vi "ts.vi"(7 "error in":errorcluster) -> (27 "error out":errorcluster)   [LabVIEW 2017]
uses:
  <vilib>/vision/NI_Vision_Development_Module.lvlib
panel:
  out "Image Out":T1(plugin-control)
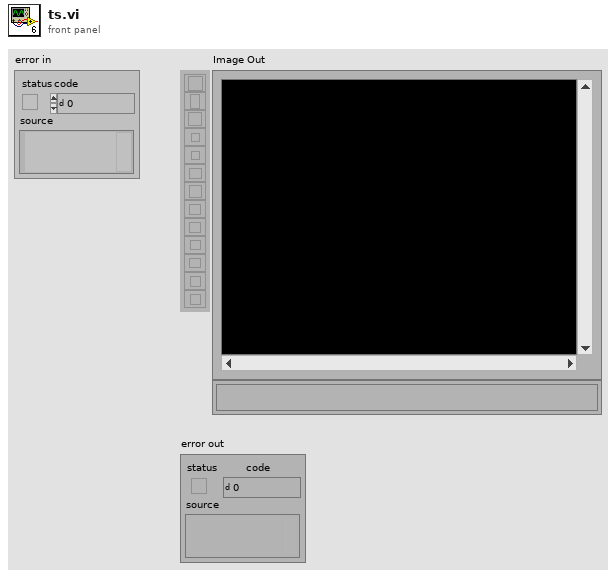
[diagram p1: front panel]
types:
  T1 = typedef "IMAQ Image.ctl" = refnum<image>
  T2 = cluster{"Origin Pixel":cluster{"X":sgl, "Y":sgl}, "Angle Relative to Horizontal (deg)":sgl, "Axis Reference":u32}
  T3 = typedef "Image Type" = u32
  T4 = cluster{"Origin Pixel":cluster{"X":sgl, "Y":sgl}, sgl, "Axis Reference":u32}
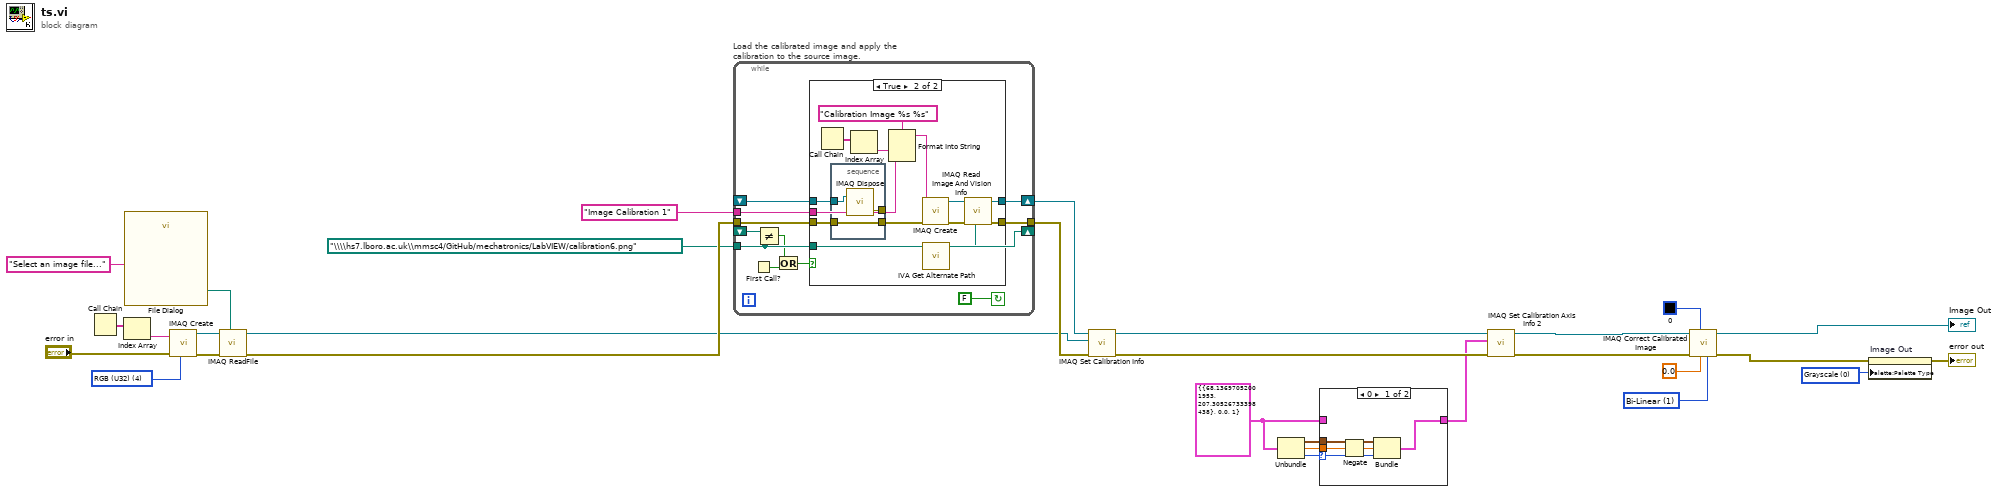
[diagram p0: block diagram]
diagram:
  w1 = u32 0 items=["Grayscale", "Binary", "Gradient", "Rainbow", "Temperature", "User Defined", "Binary 16 Bit", "Gradient 16 Bit", "Rainbow 16 Bit", "Temperature 16 Bit", "User Defined 16 Bit"] ("Palette Type")
  w8 = u32 1 items=["Zero Order", "Bi-Linear", "Quadratic", "Cubic Spline"] ("Interpolation Type")
  w12 = T2 {"Origin Pixel"={"X"=68.13697, "Y"=207.30527}, "Angle Relative to Horizontal (deg)"=0.0, "Axis Reference"=1} ("Calibration Axis Info")
  w22 = T3 4 items=["Grayscale (U8)", "Grayscale (I16)", "Grayscale (SGL)", "Complex (CSG)", "RGB (U32)", "HSL (U32)", "RGB (U64)", "Grayscale (U16)"] ("Image Type")
  n1 = Call Chain() -> (call chain=w26:string[])
  n2 = Index Array(array=w26) -> (element=w25:string)  [unwired: 1 in]
  n3 = call "File Dialog"("prompt"="Select an image file...") -> ("selected path"=w23:path)  [unwired: 6 in, 8 out]
  n4 = call "IMAQ Create"("Image Name"=w25, "Image Type"=w22, "error in (no error)"="error in") -> ("New Image"=w29:T1, "error out"=w28:errorcluster)  [unwired: 1 in, 1 out]
  n5 = call "IMAQ ReadFile"("File Path"=w23, "error in (no error)"=w28, "Image"=w29) -> ("error out"=w30:errorcluster, "Image Out"=w17:T1)  [unwired: 2 in, 5 out]
  n6 = while "Load the calibrated image and apply the calibration to the source image." {
    shift-right: [w41] -> w20
    shift-left: _ -> [w40]
    tunnel: [w38] -> w19
    tunnel: w30 -> [w37]
    tunnel: path "\\\\hs7.lboro.ac.uk\\mmsc4/GitHub/mechatronics/LabVIEW/calibration6.png" ("File Path") -> [w34]
    tunnel: "Image Calibration 1" ("Step Name") -> [w36]
    shift-right: [w34] -> _
    shift-left: _ -> [w35]
    stop <- FALSE continue-if-true
    n7 = First Call?() -> (First Call?: T/F=w33:bool)
    n8 = Not Equal?(x=w35, y=w34) -> (x != y?=w32:bool)
    n9 = Or(x=w32, y=w33) -> (x .or. y?=w31:bool)
    n10 = case shown="True" w31 {
      tunnel: [w43 w55] -> w41
      tunnel: w40 -> [w43 w47]
      tunnel: [w42 w52] -> w38
      tunnel: w37 -> [w42 w48]
      tunnel: w34 -> [_ w45]
      tunnel: w36 -> [_ w49]
      frame False {
      }
      frame True {
        n11 = Call Chain() -> (call chain=w51:string[])
        n12 = stacked-sequence {
          tunnel: w48 -> [w59]
          tunnel: w47 -> [w60]
          tunnel: [w59] -> w46
          tunnel: [w58] -> _
          frame #0 {
            n13 = call "IMAQ Dispose"("Image"=w60) -> ("error out"=w58:errorcluster)  [unwired: 2 in, 3 out]
          }
        }
        n14 = Index Array(array=w51) -> (element=w50:string)  [unwired: 1 in]
        n15 = Format Into String(format string="Calibration Image %s %s" ("Image Name"), w50, w49) -> (resulting string=w57:string)  [unwired: 2 in, 1 out]
        n16 = call "IMAQ Create"("Image Name"=w57, "error in (no error)"=w46) -> ("New Image"=w54:T1, "error out"=w53:errorcluster)  [unwired: 2 in, 1 out]
        n17 = call <vilib>:"IVA Get Alternate Path.vi"("Path In"=w45) -> ("Path Out"=w44:path)  [unwired: 10 out]
        n18 = call "IMAQ Read Image And Vision Info"("File Path"=w44, "error in (no error)"=w53, "Image"=w54) -> ("error out"=w52:errorcluster, "Image Out"=w55:T1)  [unwired: 1 in, 6 out]
      }
    }
  }
  n19 = call "IMAQ Set Calibration Info"("error in (no error)"=w19, "Image Dst"=w17, "Image Src"=w20) -> ("error out"=w18:errorcluster, "Calibrated Image"=w14:T1)  [unwired: 1 in, 6 out]
  n20 = Unbundle(w12) -> ("Origin Pixel"=w9:cluster{"X":sgl, "Y":sgl}, "Angle Relative to Horizontal (deg)"=w10:sgl, "Axis Reference"=w13:u32)
  n21 = case shown="0" w13 {
    selector: w13 -> [w62 _]
    tunnel: w12 -> [_ w66]
    tunnel: [w61 w66] -> w11
    tunnel: w10 -> [w65 _]
    tunnel: w9 -> [w64 _]
    frame 0 {
      n22 = Negate(x=w65) -> (-x=w63:sgl)
      n23 = Bundle("Origin Pixel"=w64, w63, "Axis Reference"=w62) -> (w61:T4)  [unwired: 1 in]
    }
    frame 1, Default {
    }
  }
  n24 = call-poly "IMAQ Set Calibration Axis Info 2"("error in (no error)"=w18, "Calibration Axis Info"=w11, "Calibration Template Image In"=w14) -> ("error out"=w15:errorcluster, "Calibration Template Image Out"=w6:T1)  [unwired: 7 out]
  n25 = call "IMAQ Correct Calibrated Image"("Interpolation Type"=w8, "Replace Value"=sgl 0.0, "Color Replace Value"=u32 0, "error in (no error)"=w15, "Image Src"=w6) -> ("error out"=w7:errorcluster, "Corrected Image"=→"Image Out":T1)  [unwired: 2 in, 3 out]
  n26 = property on="Image Out" class="ImageControl"(error in=w7, "Palette:Palette Type"=w1) -> (error out=→"error out":errorcluster)  [unwired: 1 in, 1 out]
